vi "button.vi"() -> ()   [LabVIEW 2017]
panel:
  in  "Add":bool
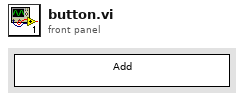
[diagram p1: front panel]
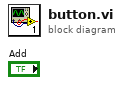
[diagram p0: block diagram]
diagram:
